vi "Old-Main.vi"() -> ()   [LabVIEW 2016]
panel:
  out "Thresholding":i16[][](graph)
  out "Red":u8[][](graph)
  out "Blue":u8[][](graph)
  out "Output":u16[][](graph)
  out "Luminousity":u8[][](graph)
  in  "Maze Path":path=path "C:/Users/Luke Jarocki/Downloads/maze_2.jpg"
  out "Value":dbl[][](graph)
  # "White"
  # "Not White"
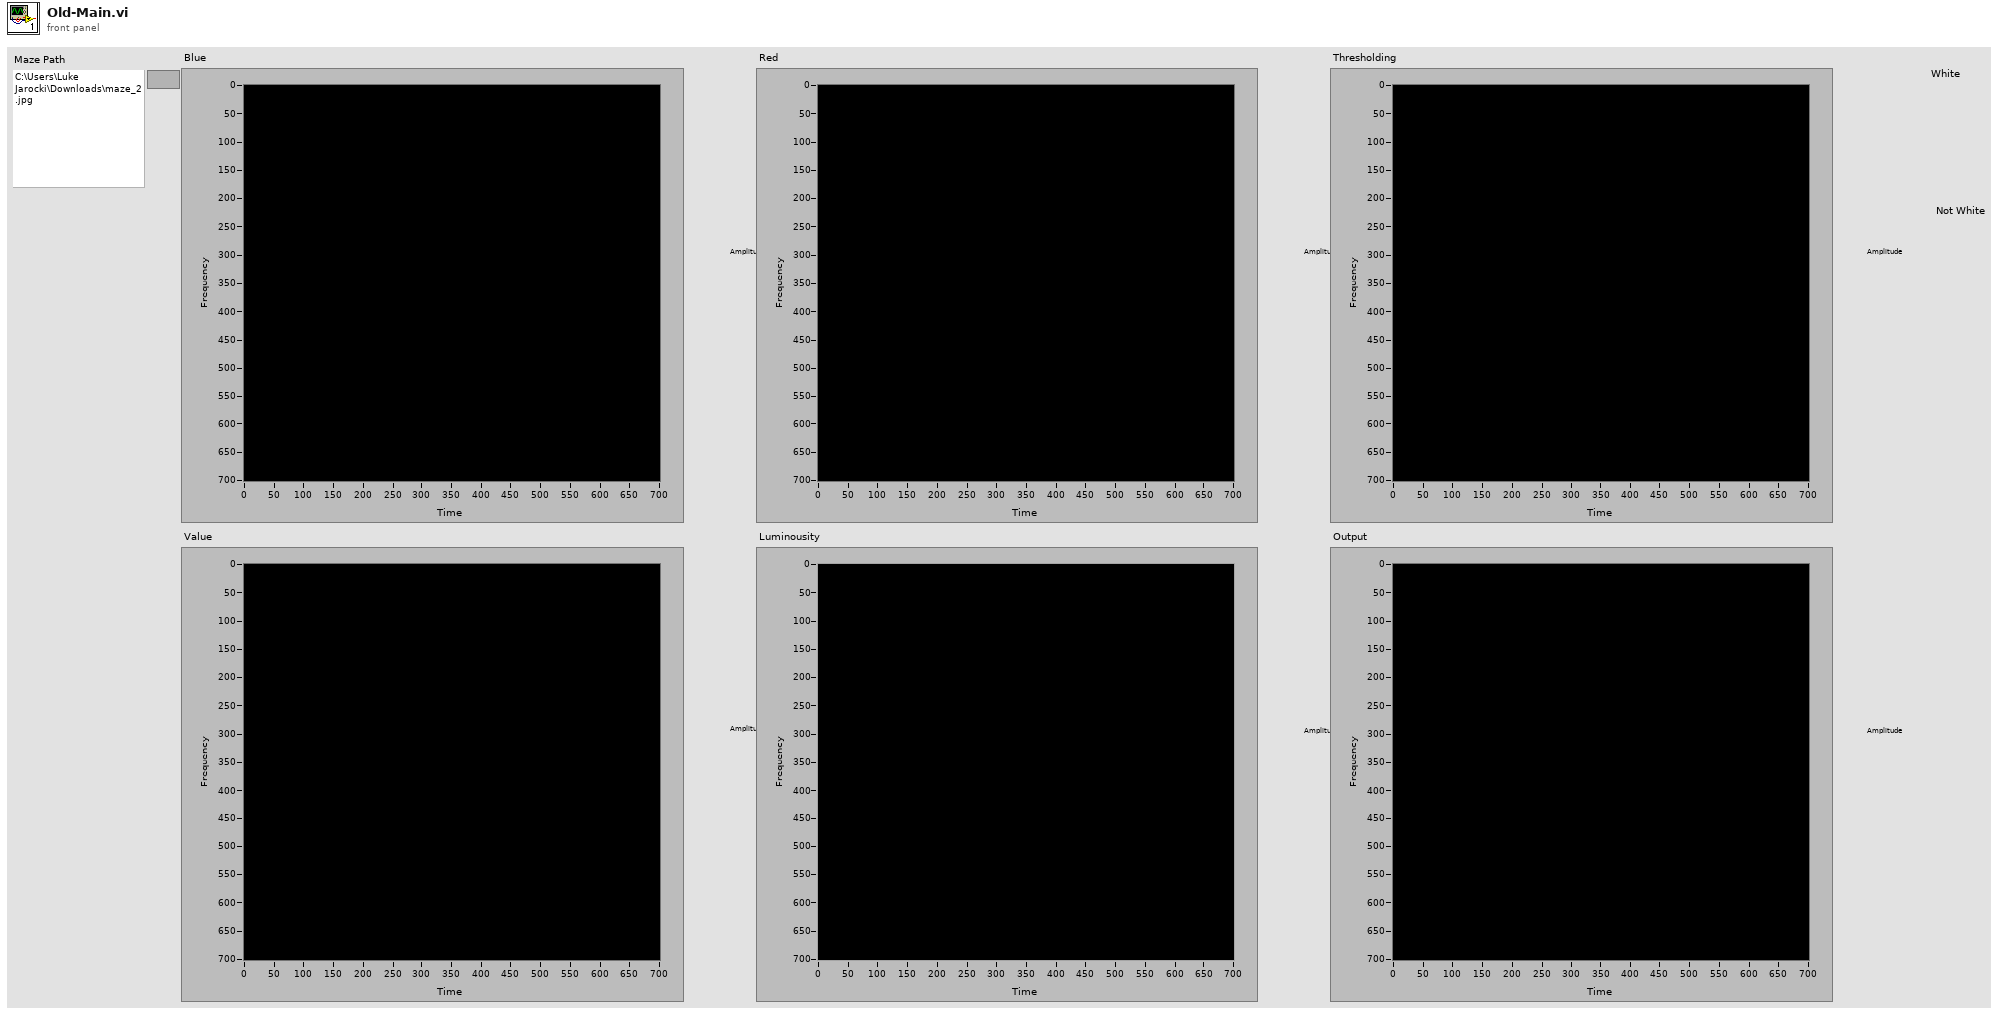
[diagram p1: front panel]
types:
  T1 = typedef "imagedata.ctl" = cluster{"image type":i32, "image depth":i32, "image":u8[], "mask":u8[], "colors":u32[], "Rectangle":cluster{"left":i16, "top":i16, "right":i16, "bottom":i16}}
  T2 = typedef "TileColor.ctl" = u16
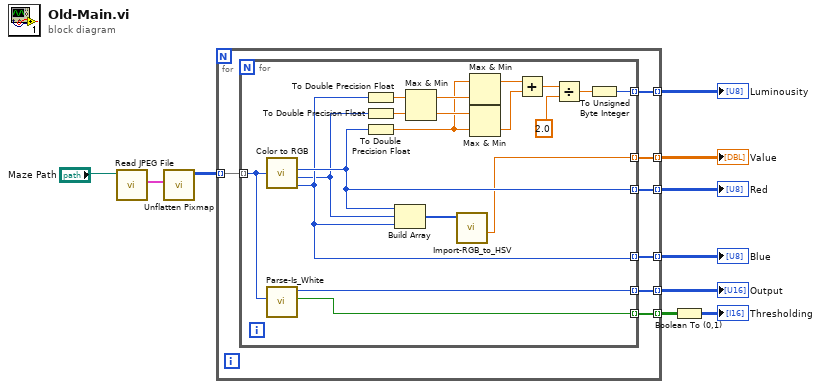
[diagram p0: block diagram]
diagram:
  n1 = call <vilib>:"Read JPEG File.vi"("path to JPEG file"="Maze Path") -> ("image data"=w10:T1)  [unwired: 8 in, 2 out]
  n2 = call <vilib>:"Unflatten Pixmap.vi"("image data"=w10) -> ("24-bit pixmap"=w1:u32[][])  [unwired: 4 in, 6 out]
  n3 = for {
    tunnel: w1 -> [w17] mode=indexing
    tunnel: [w16] -> w8 mode=indexing
    tunnel: [w15] -> w3 mode=indexing
    tunnel: [w14] -> w7 mode=indexing
    tunnel: [w13] -> w6 mode=indexing
    tunnel: [w12] -> w5 mode=indexing
    tunnel: [w11] -> w4 mode=indexing
    n4 = for {
      tunnel: w17 -> [w21] mode=indexing
      tunnel: [w22] -> w16 mode=indexing
      tunnel: [w25] -> w15 mode=indexing
      tunnel: [w26] -> w14 mode=indexing
      tunnel: [w23] -> w13 mode=indexing
      tunnel: [w20] -> w12 mode=indexing
      tunnel: [w19] -> w11 mode=indexing
      n5 = call <vilib>:"Color to RGB.vi"("Color"=w21) -> ("R"=w26:u8, "G"=w18:u8, "B"=w25:u8)  [unwired: 1 out]
      n6 = call "Parse-Is_White.vi"("Color"=w21) -> ("Is White"=w19:bool, "Tile Color"=w20:T2)  [unwired: 8 in, 1 out]
      n7 = To Double Precision Float(number=w25) -> (double precision float=w30:dbl)
      n8 = To Double Precision Float(number=w18) -> (double precision float=w29:dbl)
      n9 = To Double Precision Float(number=w26) -> (double precision float=w27:dbl)
      n10 = Build Array(w26, w18, w25) -> (w24:u8[])
      n11 = Max & Min(x=w30, y=w29) -> (max(x,y)=w35:dbl, min(x,y)=w36:dbl)
      n12 = call "Import-RGB_to_HSV.vi"("RGB"=w24) -> ("Value"=w23:dbl)  [unwired: 7 in, 3 out]
      n13 = Max & Min(x=w27, y=w35) -> (max(x,y)=w34:dbl)  [unwired: 1 out]
      n14 = Max & Min(x=w36, y=w27) -> (min(x,y)=w33:dbl)  [unwired: 1 out]
      n15 = Add(x=w34, y=w33) -> (x+y=w32:dbl)
      n16 = Divide(x=w32, y=2.0) -> (x/y=w28:dbl)
      n17 = To Unsigned Byte Integer(number=w28) -> (unsigned 8bit integer=w22:u8)
    }
  }
  "Luminousity" <- w8
  "Red" <- w7
  "Output" <- w5
  "Blue" <- w3
  "Value" <- w6
  n18 = Boolean To (0,1)(Boolean=w4) -> (0, 1=→"Thresholding":i16[][])
